vi "Create NT Scalar (NT Base).vi"(8 "error in (no error)":errorcluster, 9 "fields":T1, 10 "initial value":refnum<class "NT Scalar.lvclass">) -> (0 "error out":errorcluster, 2 "value out":refnum<class "NT Scalar.lvclass">, 3 "PV Data out":refnum<class "PV Data.lvclass">)   [LabVIEW 2020, in "PV Access.lvlib" / "PV Data.lvlib" / "PV Data.lvclass"]
uses:
  PV Data.lvclass
  NT Scalar/NT Scalar.lvclass
  C:/Users/eyw68381/source/repos/pvaccess-labview/labview/source/PV Data/NT Base/NT Base.lvclass
  PV Data.lvclass/PV Data.ctl
  Value Fields.ctl
  PV Data.lvlib
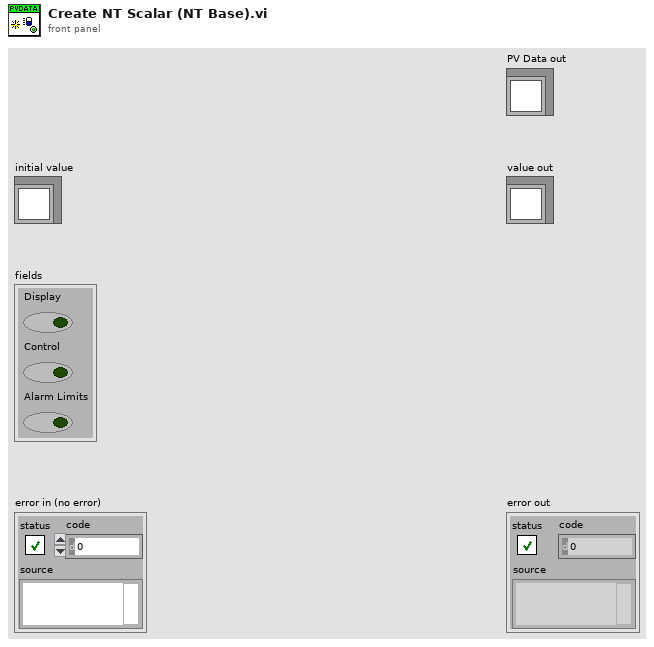
[diagram p1: front panel]
types:
  T1 = typedef "PV Access.lvlib/PV Data.lvlib/Value Fields.ctl" = cluster{"Display":bool, "Control":bool, "Alarm Limits":bool}
  T2 = typedef "PV Access.lvlib/PV Data.lvlib/Type Code.ctl" = enum8{"Null", "Bool", "BoolA", "Int8", "Int8A", "Int16", "Int16A", "Int32", "Int32A", "Int64", "Int64A", "UInt8", "UInt8A", "UInt16", "UInt16A", "UInt32", "UInt32A", "UInt64", "UInt64A", "Float32", "Float32A", "Float64", "Float64A", "String", "StringA", "Struct", "StructA", "Union", "UnionA", "Any", "AnyA"}
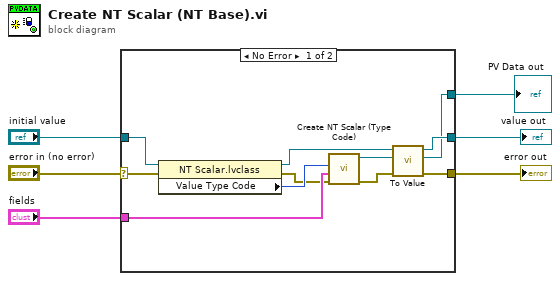
[diagram p0: block diagram]
diagram:
  n1 = case shown="No Error" "error in (no error)" {
    selector: "error in (no error)" -> [w17 w18]
    tunnel: "fields" -> [w16 _]
    tunnel: "initial value" -> [w15 w19]
    tunnel: [w14 w18] -> w3
    tunnel: [w13 w19] -> w2
    tunnel: [w12 _] -> w1
    frame No Error {
      n2 = property class="NT Scalar.lvclass"(reference=w15, error in=w17) -> (reference out=w7:refnum<class "NT Scalar.lvclass">, error out=w9:errorcluster, "Value Type Code"=w10:T2)
      n3 = call "Create NT Scalar (Type Code).vi"("error in"=w9, "value fields"=w16, "type code"=w10) -> ("error out"=w11:errorcluster, "PV Data out"=w8:refnum<class "PV Data.lvclass">)  [unwired: 7 in]
      n4 = call-dynamic "To Value.vi"("error in (no error)"=w11, "PV Data in"=w8, "NTBase in"=w7) -> ("error out"=w14:errorcluster, "PV Data out"=w12:refnum<class "PV Data.lvclass">, "NTBase out"=w13:refnum<class "NT Scalar.lvclass">)  [unwired: 6 in]
    }
    frame Error {
    }
  }
  "error out" <- w3
  "PV Data out" <- w1
  "value out" <- w2
